vi "Get GOOP Refnum.vi"(11 "LabVIEW Object in":refnum<class>) -> (0 "No Levels a GOOP obj":bool, 1 "Not a Ref Yet?":bool, 2 "Not Goop by Level":bool[](array[boolean]), 3 "Refnum?":u32[](array[numeric]))   [LabVIEW 2019, in "GOOP Probe.lvlib"]
uses:
  GOOP Probe.lvlib
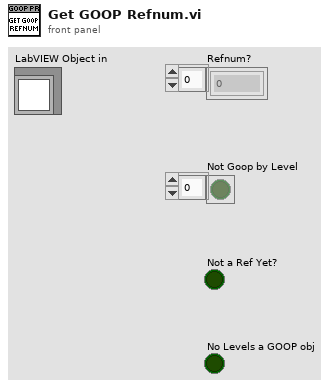
[diagram p1: front panel]
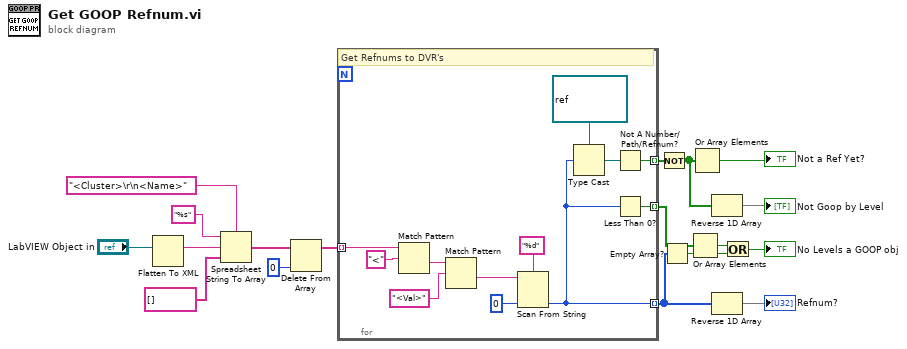
[diagram p0: block diagram]
diagram:
  n1 = Flatten To XML(anything="LabVIEW Object in") -> (xml string=w14:string)
  n2 = Spreadsheet String To Array(delimiter (Tab)="<Cluster>\r\n<Name>", format string="%s", spreadsheet string=w14, array type (2D Dbl)=string[] []) -> (array=w12:string[])
  n3 = Delete From Array(array=w12, index=0) -> (array with subset deleted=w13:string[])  [unwired: 1 in, 1 out]
  n4 = for {
    tunnel: w13 -> [w30] mode=indexing
    tunnel: [w21] -> w9 mode=indexing
    tunnel: [w20] -> w6 mode=indexing
    tunnel: [w19] -> w3 mode=indexing
    # "Get Refnums to DVR's"
    n5 = Match Pattern(string=w30, regular expression="<") -> (after substring=w24:string)  [unwired: 1 in, 3 out]
    n6 = Match Pattern(string=w24, regular expression="<Val>") -> (after substring=w25:string)  [unwired: 1 in, 3 out]
    n7 = Scan From String(format string="%d", input string=w25, default 1=u32 0 ("default value 1")) -> (output 1=w21:u32)  [unwired: 2 in, 3 out]
    n8 = Type Cast(type=refnum<data-value> refnum ("data value reference"), x=w21) -> (*(type *) &x=w22:refnum<data-value>)
    n9 = Not A Number/Path/Refnum?(number/path/refnum=w22) -> (NaN/Path/Refnum?=w19:bool)
    n10 = Less Than 0?(x=w21) -> (x < 0?=w20:bool)
  }
  n11 = Not(x=w3) -> (.not. x?=w1:bool[])
  n12 = Empty Array?(array=w9) -> (empty?=w4:bool)
  n13 = Or Array Elements(Boolean array=w6) -> (logical OR=w5:bool)
  n14 = Or Array Elements(Boolean array=w1) -> (logical OR=→"Not a Ref Yet?":bool)
  n15 = Reverse 1D Array(array=w1) -> (reversed array=→"Not Goop by Level":bool[])
  n16 = Reverse 1D Array(array=w9) -> (reversed array=→"Refnum?":u32[])
  n17 = Or(x=w5, y=w4) -> (x .or. y?=→"No Levels a GOOP obj":bool)
